vi "ConvertPercentVbusToVoltage.vi"(11 "Vbus":dbl) -> (3 "Voltage":dbl)   [LabVIEW 2015]
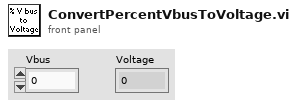
[diagram p1: front panel]
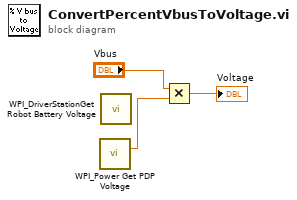
[diagram p0: block diagram]
diagram:
  n1 = call <vilib>:"WPI_Power Get PDP Voltage.vi"() -> ("voltage (V)"=w1:dbl)  [unwired: 14 in, 1 out]
  n2 = call <vilib>:"WPI_DriverStationGet Robot Battery Voltage.vi"() -> ()  [unwired: 14 in, 2 out]
  n3 = Multiply(x="Vbus", y=w1) -> (x*y=→"Voltage":dbl)
